vi "Text_Convolutional_test.vi"() -> ()   [LabVIEW 2014]
uses:
  <vilib>/addons/Modulation/Digital/Channel Coding/MT Convolutional Encoder (Rate).vi
  <vilib>/addons/Modulation/Digital/Support/Common/Validators/mod_Validate Bit Stream.vi
  <vilib>/addons/Modulation/Digital/Channel Coding/Convolutional codes/mod_Convolutional encoder.vi
  <vilib>/addons/Modulation/Analog/support/mod_Set Error Source.vi
  <vilib>/addons/Modulation/Digital/Channel Coding/Convolutional codes/subVIs/mod_Generate encoder tap connections.vi
  <vilib>/addons/Modulation/Digital/Channel Coding/Convolutional codes/subVIs/mod_Perform convolutional encoding.vi
  <vilib>/addons/Modulation/Digital/Channel Coding/Block codes/subVIs/mod_Buffer block code info (I8).vi
  <vilib>/addons/Modulation/Digital/Channel Coding/Convolutional codes/subVIs/mod_Generate valid reset (convolutional, I8).vi
  <vilib>/addons/Modulation/Digital/Channel Coding/Convolutional codes/subVIs/mod_Select known generator matrix.vi
  <vilib>/addons/Modulation/Digital/Support/Common/Validators/mod_Validate Convolutional Encoder prms.vi
  <vilib>/addons/Modulation/Digital/Channel Coding/MT Convolutional Decoder (Viterbi Hard Decision, Rate).vi
  <vilib>/addons/Modulation/niDMT.lvlib
panel:
  out "final state":u32 format="%.0x"
  out "output bit stream 3":i8[](array[numeric])
  out "error out":errorcluster
  out "output bit stream":i8[](array[numeric])
  in  "constraint length (K)":i32=3
  in  "rate (k/n)":enum16{"1/2", "1/3", "1/4", "2/3", "3/4"}(ring)
  out "string":string
  out "Number of Packets":i32
  in  "Packet\nMessage Length (bits)":i32
  in  "text":string
  out "output bit stream 2":i8[](array[numeric]) caption="output bit stream"
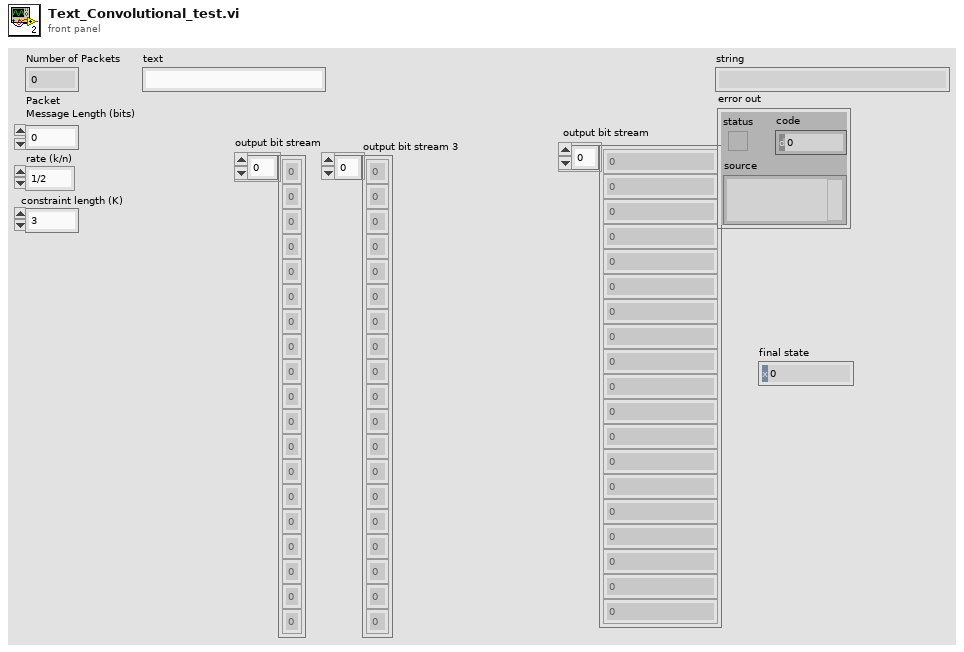
[diagram p1: front panel]
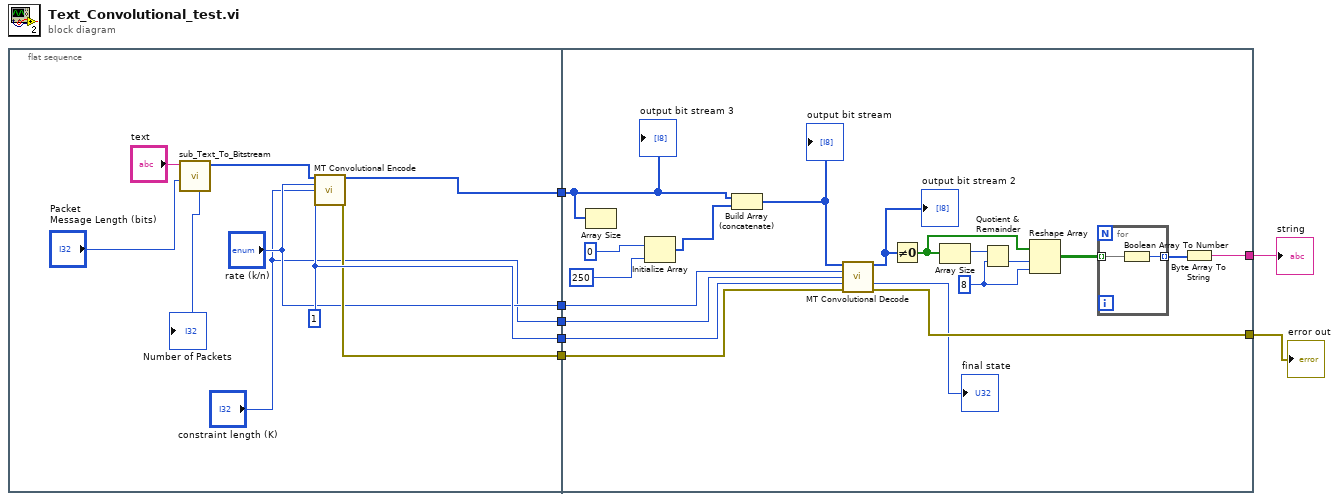
[diagram p0: block diagram]
diagram:
  n1 = flat-sequence {
    tunnel: ["constraint length (K)"] -> w7
    tunnel: [w13] -> w6
    tunnel: [w12] -> w5
    tunnel: [w11] -> w2
    tunnel: ["rate (k/n)"] -> w1
    tunnel: w7 -> [w23]
    tunnel: w6 -> [w24]
    tunnel: w5 -> [w25]
    tunnel: [w27] -> w4
    tunnel: [w26] -> w3
    tunnel: w2 -> [w22]
    tunnel: w1 -> [w29]
    frame #0 {
      w13 = u32 1 ("initial state")
      n2 = call "sub_Text_To_Bitstream.vi"("Packet\nMessage Length (bits)"="Packet\nMessage Length (bits)", "text"="text") -> ("message bitstream"=w8:i8[], "Number of Packets"=→"Number of Packets":i32)  [unwired: 7 in, 1 out]
      n3 = call-poly <vilib>:"MT Convolutional Encode.vi"("input bit stream"=w8, "rate (k/n)"="rate (k/n)", "constraint length (K)"="constraint length (K)", "initial state"=w13) -> ("output bit stream"=w11:i8[], "error out"=w12:errorcluster)  [unwired: 9 in, 1 out]
    }
    frame #1 {
      w33 = 8
      n4 = Array Size(array=w22) -> ()  [unwired: 1 out]
      n5 = Initialize Array(0, 250 ("dimension size")) -> (w18:i32[])
      n6 = Build Array (concatenate)(w22, w18) -> (w21:i32[])
      "output bit stream" <- w21
      n7 = call-poly <vilib>:"MT Convolutional Decode.vi"("input bit stream"=w21, "rate (k/n)"=w29, "constraint length (K)"=w23, "initial state"=w24, "error in (no error)"=w25) -> ("output bit stream"=w28:i8[], "final state"=→"final state":u32, "error out"=w26:errorcluster)  [unwired: 8 in]
      "output bit stream 2" <- w28
      n8 = Not Equal To 0?(x=w28) -> (x != 0?=w31:bool[])
      n9 = Array Size(array=w31) -> (size(s)=w32:i32)
      n10 = Quotient & Remainder(x=w32, y=w33) -> (floor(x/y)=w34:i32)  [unwired: 1 out]
      n11 = Reshape Array(w31, w34, w33) -> (w30:bool[][])
      n12 = for {
        tunnel: [w37] -> w35 mode=indexing
        tunnel: w30 -> [w36] mode=indexing
        n13 = Boolean Array To Number(Boolean array=w36) -> (number=w37:u32)
      }
      n14 = Byte Array To String(unsigned byte array=w35) -> (string=w27:string)
      "output bit stream 3" <- w22
    }
  }
  "string" <- w4
  "error out" <- w3
